vi "Bajada.vi"(8 "thetaf":dbl, 10 "thetai":dbl) -> (2 "dt":dbl)   [LabVIEW 2018]
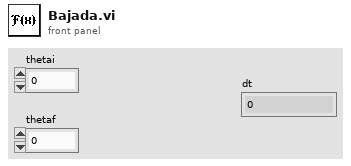
[diagram p1: front panel]
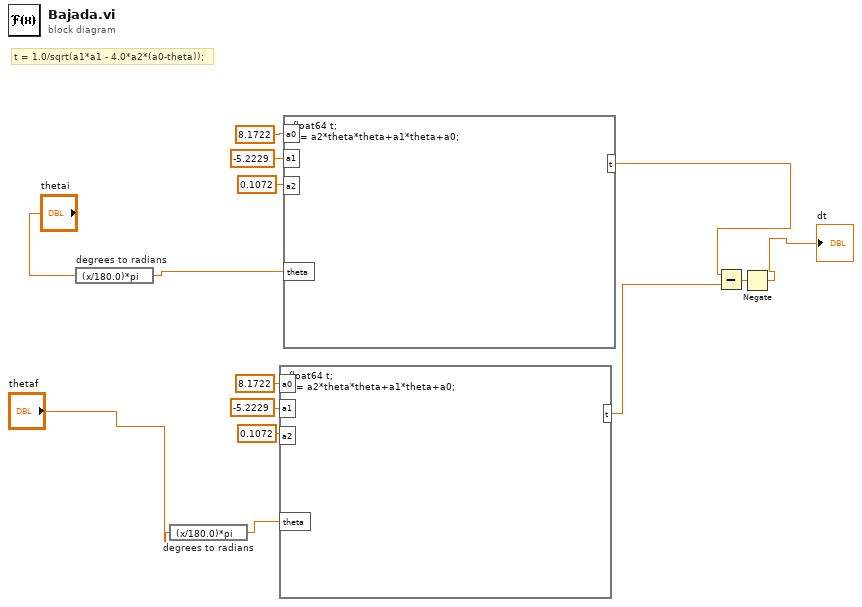
[diagram p0: block diagram]
diagram:
  # "t = 1.0/sqrt(a1*a1 - 4.0*a2*(a0-theta));"
  n1 = expression code="(x/180.0)*pi" "degrees to radians"("thetai") -> (w10:dbl)
  n2 = expression code="(x/180.0)*pi" "degrees to radians"("thetaf") -> (w2:dbl)
  n3 = formula code="float64 t;\nt = a2*theta*theta+a1*theta+a0;"("a0"=8.1722 ("input variable"), "a1"=-5.2229 ("input variable"), "a2"=0.1072 ("input variable"), "theta"=w2) -> ("t"=w1:dbl)
  n4 = formula code="float64 t;\nt = a2*theta*theta+a1*theta+a0;"("a0"=8.1722 ("input variable"), "a1"=-5.2229 ("input variable"), "a2"=0.1072 ("input variable"), "theta"=w10) -> ("t"=w8:dbl)
  n5 = Subtract(x=w8, y=w1) -> (x-y=w7:dbl)
  n6 = Negate(x=w7) -> (-x=→"dt":dbl)
